vi "PH_PSDBWriter.PC Write PSDB.vi"(0 "i ref in":refnum<vi>, 5 "error IO":errorcluster) -> (14 "i ref out":refnum<vi>, 19 "error out":errorcluster)   [LabVIEW 2014, in "PH_PSDBWriter.lvlib"]
doc: "This is the proc case which writes data to the PHELIX shot data base."
uses:
  PH_PSDBWriter.lvlib
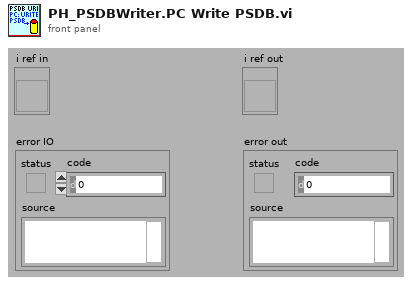
[diagram p1: front panel]
types:
  T1 = typedef "PH_PSDBWriter.lvlib/PH_PSDBWriter.Data Status.ctl" = i16
  T2 = typedef "PH_PSDBWriter.lvlib/PH_PSDBWriter.i attribute.ctl" = cluster{"PSDB Status Service ID":i32, "Instance ID":i32, "Shot #":i32, "Subsystem":T3, "Data Status":T1, "Ref PSDB Status":refnum<vi>, "PSDB Error Code":i32, "PSDB Dataset":T4, "PSDB Thread":cluster{"Ref":refnum<vi>, "Q-Ref":refnum<queue>}, "PSDB Credentials":T12}
  T3 = typedef "PH_PSDBWriter.lvlib/PH_PSDBWriter.PHELIX-Subsystems.ctl" = i32
  T4 = typedef "PH_PSDBWriter.lvlib/PH_PSDBWriter.PSDB Dataset.ctl" = cluster{"Version":i32, "2D data Input":T5[], "Boolean Input":T7[], "Image Input":T8[], "Numeric Input":T10[], "String Input":T11[]}
  T5 = typedef "PH_PSDBWriter.lvlib/PH_PSDBWriter.2D dataset.ctl" = cluster{"name":string, "data":dbl[][], "axis description":T6}
  T6 = typedef "PSDB.lvlib/PSDB_AxisDescription.ctl" = cluster{"x axis label":string, "y axis label":string, "x axis unit":string, "y axis unit":string}
  T7 = typedef "PH_PSDBWriter.lvlib/PH_PSDBWriter.Boolean dataset.ctl" = cluster{"name":string, "data":bool, "unit":string}
  T8 = typedef "PH_PSDBWriter.lvlib/PH_PSDBWriter.Image dataset.ctl" = cluster{"name":string, "data":T9, "unit":string}
  T9 = typedef "IMAQ Image.ctl" = refnum<image>
  T10 = typedef "PH_PSDBWriter.lvlib/PH_PSDBWriter.Numeric dataset.ctl" = cluster{"name":string, "data":dbl, "unit":string}
  T11 = typedef "PH_PSDBWriter.lvlib/PH_PSDBWriter.String dataset.ctl" = cluster{"name":string, "data":string, "unit":string}
  T12 = typedef "PH_Common.lvlib/PH_Connection.PSDB Credentials.ctl" = cluster{"PW":string, "ID":string, "DS":string}
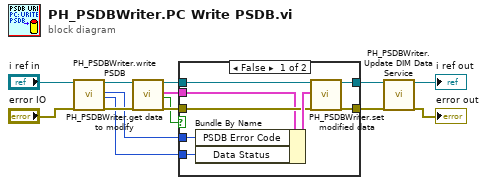
[diagram p0: block diagram]
diagram:
  n1 = call "PH_PSDBWriter.write PSDB.vi"("VI in"="i ref in", "error in"="error IO") -> ("VI out"=w4:refnum<vi>, "PSDB Error code"=w6:i32, "Data Status"=w7:T1, "error out"=w8:errorcluster)  [unwired: 14 in]
  n2 = call "PH_PSDBWriter.get data to modify.vi"("i ref in"=w4, "error in (no error)"=w8) -> ("i ref out"=w3:refnum<vi>, "i attribute"=w2:T2, "timed out"=w1:bool, "error out"=w5:errorcluster)  [unwired: 14 in]
  n3 = case shown="False" w1 {
    tunnel: [w22 w24] -> w11
    tunnel: [w21 w23] -> w9
    tunnel: w7 -> [w20 _]
    tunnel: w6 -> [w18 _]
    tunnel: w5 -> [w17 w23]
    tunnel: w3 -> [w16 w24]
    tunnel: w2 -> [w15 _]
    frame False {
      n4 = Bundle By Name(cluster=w15, "PSDB Error Code"=w18, "Data Status"=w20) -> (w19:T2)
      n5 = call "PH_PSDBWriter.set modified data.vi"("i ref in"=w16, "i attribute"=w19, "error in (no error)"=w17) -> ("i ref out"=w22:refnum<vi>, "error out"=w21:errorcluster)  [unwired: 15 in]
    }
    frame True {
    }
  }
  n6 = call "PH_PSDBWriter.Update DIM Data Service.vi"("i ref in"=w11, "error in"=w9) -> ("i ref out"=→"i ref out":refnum<vi>, "error out"=→"error out":errorcluster)  [unwired: 16 in]
